vi "WriteConfig.vi"(3 "error in":errorcluster, 4 "Value":string[](array[string]), 5 "section":string) -> (0 "error out":errorcluster)   [LabVIEW 2015]
uses:
  <vilib>/Utility/config.llb/Write Key (String).vi
  <vilib>/Utility/config.llb/NI_LVConfig.lvlib
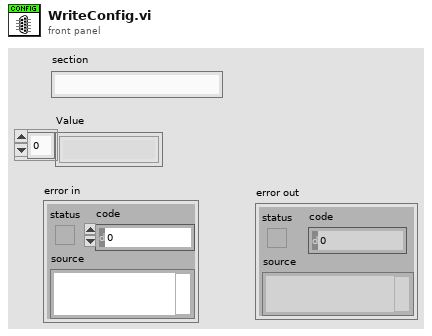
[diagram p1: front panel]
types:
  T1 = typedef "NI_LVConfig.lvlib/Config Data RefNum.ctl" = refnum<k1>
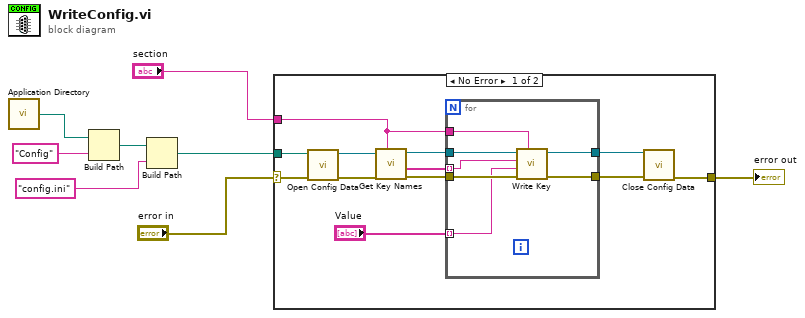
[diagram p0: block diagram]
diagram:
  n1 = call <vilib>:"Application Directory.vi"() -> ("Application Directory"=w1:path)
  n2 = Build Path(base path=w1, name or relative path="Config") -> (appended path=w3:path)
  n3 = Build Path(base path=w3, name or relative path="config.ini" ("config File")) -> (appended path=w6:path)
  n4 = case shown="No Error" "error in" {
    selector: "error in" -> [w10 w28]
    tunnel: w6 -> [w20 _]
    tunnel: "section" -> [w14 _]
    tunnel: [w11 w28] -> w4
    frame No Error {
      n5 = call <vilib>:"Open Config Data.vi"("error in (no error)"=w10, "configuration file path"=w20) -> ("error out"=w18:errorcluster, "refnum"=w19:T1)  [unwired: 7 in, 1 out]
      n6 = call <vilib>:"Get Key Names.vi"("section"=w14, "error in (no error)"=w18, "refnum"=w19) -> ("error out"=w15:errorcluster, "key names"=w17:string[], "refnum out"=w16:T1)  [unwired: 5 in, 1 out]
      n7 = for {
        tunnel: w17 -> [w22] mode=indexing
        tunnel: w16 -> [w27]
        tunnel: w15 -> [w26]
        tunnel: w14 -> [w25]
        tunnel: [w24] -> w13
        tunnel: [w23] -> w12
        tunnel: "Value" -> [w21] mode=indexing
        n8 = call-poly <vilib>:"Write Key.vi"("section"=w25, "error in (no error)"=w26, "value"=w21, "key"=w22, "refnum"=w27) -> ("error out"=w23:errorcluster, "refnum out"=w24:T1)  [unwired: 4 in, 1 out]
      }
      n9 = call <vilib>:"Close Config Data.vi"("error in (no error)"=w12, "refnum"=w13) -> ("error out"=w11:errorcluster)  [unwired: 8 in, 1 out]
    }
    frame Error {
    }
  }
  "error out" <- w4
